vi "Main.vi"() -> ()   [LabVIEW 2013]
uses:
  Controls/Function.ctl
panel:
  out "Data":string[][](array[string])
  in  "Clear":bool
  out "Enum":T1=enum."Initialize"
  out "XY Graph 5":cluster{dbl[], dbl[]}[](graph)
  in  "Path":path=path "C:/Project/Plotter/Data/Plot Configuration.txt"
  in  "Stop":bool
  in  "Plot Chart":bool
  in  "Read INI File":bool
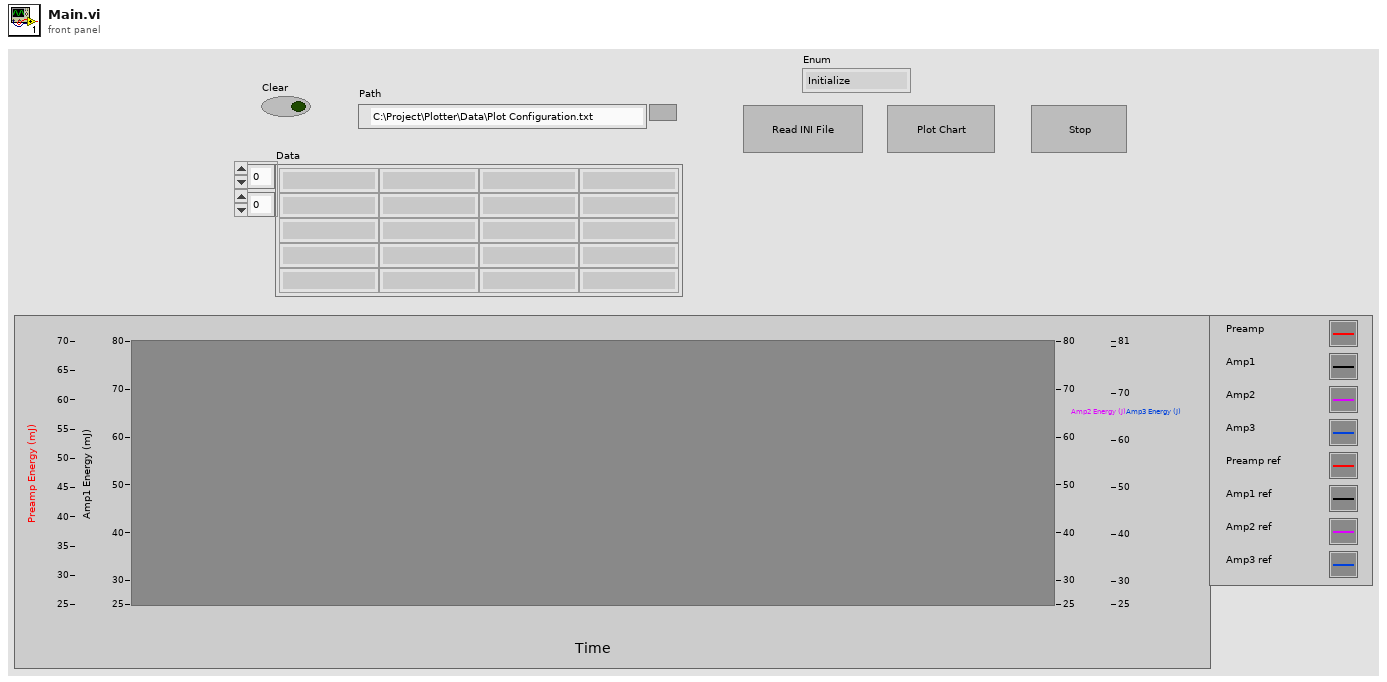
[diagram p1: front panel]
types:
  T1 = typedef "Function.ctl" = enum16{"Timeout", "Initialize", "Read INI File", "Select all variables", "Plot", "Stop"}
  T2 = cluster{"Data":string[][], "Display Names":string[], "Available Devices":string[], "References":string[]}
  T3 = cluster{"value 1":dbl, "value 2":dbl, "value 3":dbl, "value 4":dbl, "ref 1":dbl, "ref 2":dbl, "ref 3":dbl, "ref 4":dbl}
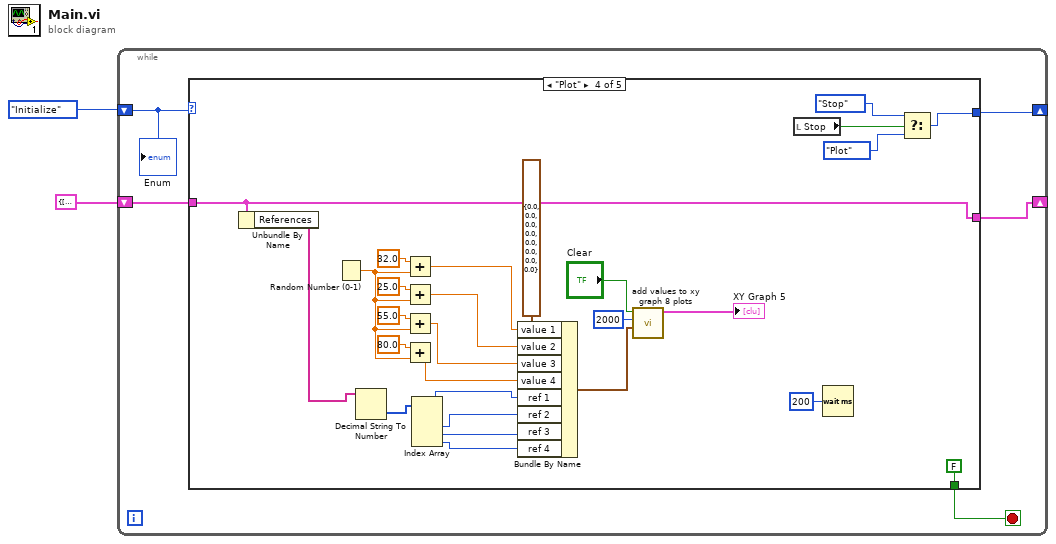
[diagram p0: block diagram]
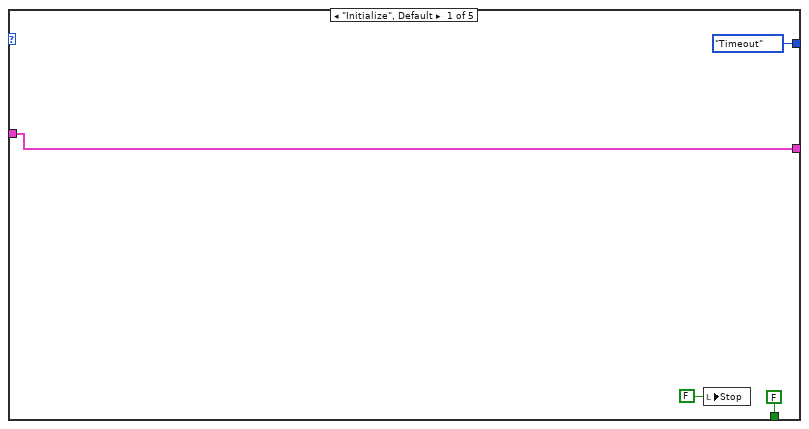
[diagram p2: hidden frame]
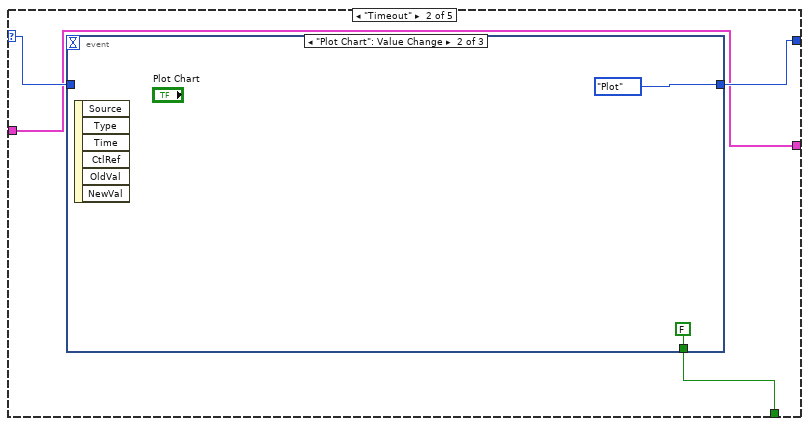
[diagram p3: hidden frame]
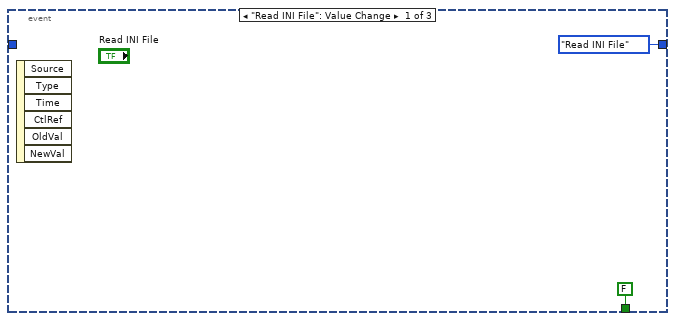
[diagram p4: hidden frame]
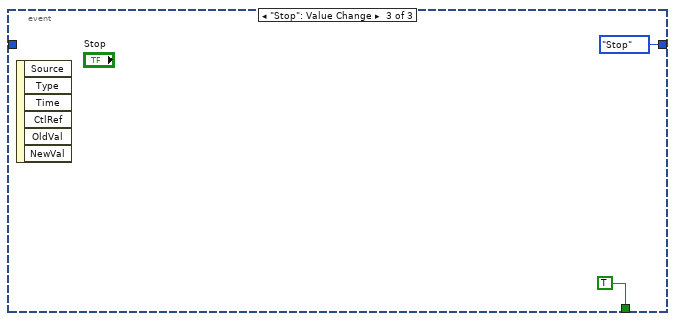
[diagram p5: hidden frame]
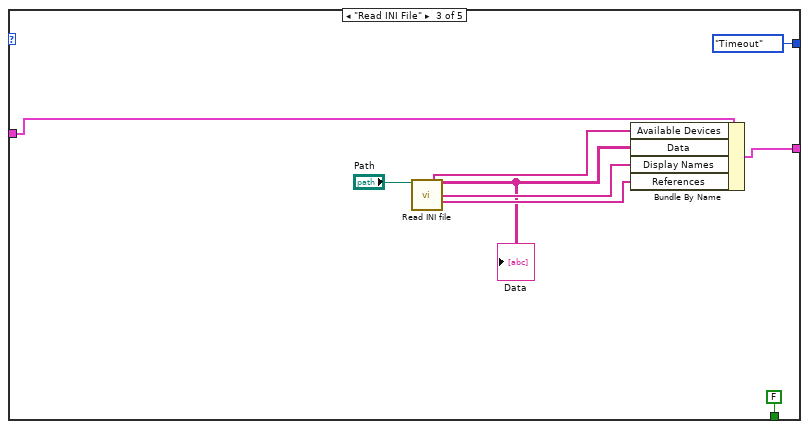
[diagram p6: hidden frame]
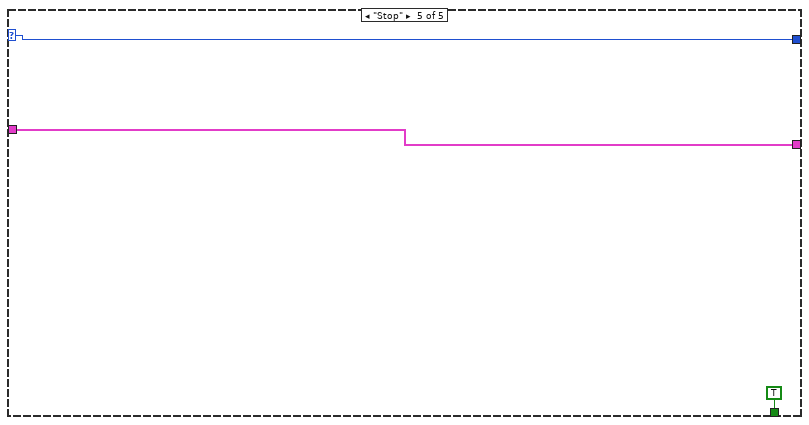
[diagram p7: hidden frame]
diagram:
  n1 = while {
    shift-right: [w7] -> _
    shift-left: Function."Initialize" -> [w6]
    shift-right: [w4] -> _
    shift-left: T2 {"Data"=[], "Display Names"=[], "Available Devices"=[], "References"=[]} -> [w3]
    stop <- w5 stop-if-true
    n2 = case shown="\"Plot\"" w6 {
      selector: w6 -> [_ w14 _ _ w60]
      tunnel: [Function."Timeout" w15 Function."Timeout" w34 w60] -> w7
      tunnel: [FALSE w13 FALSE FALSE TRUE] -> w5
      tunnel: [w11 w12 w28 w50 w58] -> w4
      tunnel: w3 -> [w11 w12 w27 w50 w58]
      frame "Initialize", Default {
        n3 = local write "Stop"(FALSE ("Stop")) -> ()
      }
      frame "Timeout" {
        n4 = event shown="[1] \"Plot Chart\": Value Change" {
          selector: _ -> [_ _ _]
          dyn-events: _ -> [_ _ _]
          timeout: _ -> [_ _ _]
          tunnel: [Function."Read INI File" Function."Plot" Function."Stop"] -> w15
          tunnel: w14 -> [_ _ _]
          tunnel: [FALSE FALSE TRUE] -> w13
          event "Read INI File": Value Change {
            n5 = event-data() -> ()  [unwired: 1 in, 6 out]
          }
          event "Plot Chart": Value Change {
            n6 = event-data() -> ()  [unwired: 1 in, 6 out]
          }
          event "Stop": Value Change {
            n7 = event-data() -> ()  [unwired: 1 in, 6 out]
          }
        }
      }
      frame "Read INI File" {
        n8 = call "Read INI file.vi"("Path"="Path") -> ("Available Devices"=w23:string[], "Data"=w24:string[][], "Display Names"=w25:string[], "References"=w26:string[])  [unwired: 9 in, 2 out]
        "Data" <- w24
        n9 = Bundle By Name(cluster=w27, "Available Devices"=w23, "Data"=w24, "Display Names"=w25, "References"=w26) -> (w28:T2)
      }
      frame "Plot" {
        n10 = Unbundle By Name(w50) -> ("References"=w51:string[])
        n11 = Random Number (0-1)() -> (number: 0 to 1=w52:dbl)
        n12 = Decimal String To Number(string=w51) -> (number=w46:i32[])  [unwired: 2 in, 1 out]
        n13 = Add(x=32.0, y=w52) -> (x+y=w38:dbl)
        n14 = Add(x=25.0, y=w52) -> (x+y=w39:dbl)
        n15 = Add(x=55.0, y=w52) -> (x+y=w40:dbl)
        n16 = Add(x=80.0, y=w52) -> (x+y=w41:dbl)
        n17 = Index Array(array=w46) -> (element #1=w42:i32, element #2=w43:i32, element #3=w44:i32, element #4=w45:i32)  [unwired: 4 in]
        n18 = Bundle By Name(cluster=T3 {"value 1"=0.0, "value 2"=0.0, "value 3"=0.0, "value 4"=0.0, "ref 1"=0.0, "ref 2"=0.0, "ref 3"=0.0, "ref 4"=0.0} ("inputs"), "value 1"=w38, "value 2"=w39, "value 3"=w40, "value 4"=w41, "ref 1"=w42, "ref 2"=w43, "ref 3"=w44, "ref 4"=w45) -> (w37:T3)
        n19 = call "add values to xy graph 8 plots.vi"("inputs"=w37, "max # points"=2000, "Clear"="Clear") -> ("xy graph"=→"XY Graph 5":cluster{dbl[], dbl[]}[])  [unwired: 8 in]
        n20 = local read "Stop"() -> (w33:bool)
        n21 = Wait (ms)(milliseconds to wait=u32 200) -> ()  [unwired: 1 out]
        n22 = Select(t=Function."Stop", s=w33, f=Function."Plot") -> (s? t:f=w34:T1)
      }
      frame "Stop" {
      }
    }
    "Enum" <- w6
  }
